vi "Emballage_NumSerie.vi"(8 "Error in":errorcluster caption="Error in (no error)", 11 "Tableau n° valves":string[](array[string])) -> (0 "Error out":errorcluster)   [LabVIEW 2020]
uses:
  Modules/FS/60_FS_Controles/60_FS_SetGet.ctl
panel:
  # "Veuillez patienter\npendant la création des fichiers \"Numéros de Série\"\nMERCI"
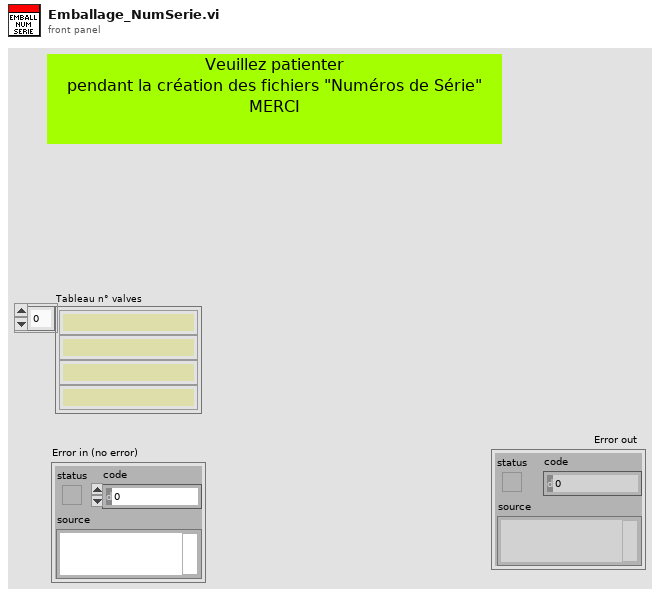
[diagram p1: front panel]
types:
  T1 = typedef "60_FS_SetGet.ctl" = enum16{"set", "get"}
  T2 = typedef "Emballage_BDD_param_Produit.ctl" = cluster{"No_Valve_FAS":string, "suffixe":string, "designation":string, "indice_produit":string, "code_barre_fixe":string, "affiche_code_barre_client":string, "affiche_no_client":string, "Nb_vlve_par_carton":u16, "melange_des_lots_possible":string, "id_article":string, "Indice_Rev":string, "Famille":string, "date":string, "code_barre_fixe_Fin":string, "Longeur_No_Serie":string}
  T3 = typedef "DATA commande.ctl" = cluster{"n°article FAS":string, "n° cmde FAS":string, "quantité cmde":string, "ID LIG cmde":string, "n° cmde client":string, "nom client":string, "n° article client":string, "indice revision client":string, "société de facturation":string, "langue a utiliser":string}
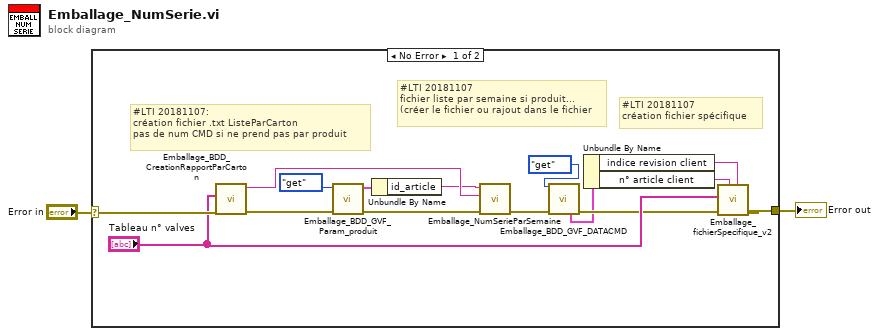
[diagram p0: block diagram]
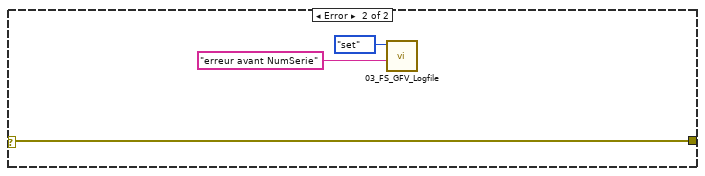
[diagram p2: hidden frame]
diagram:
  n1 = case shown="No Error" "Error in" {
    selector: "Error in" -> [w10 w18]
    tunnel: [w9 w18] -> w1
    frame No Error {
      # "#LTI 20181107\ncréation fichier spécifique"
      # "#LTI 20181107\nfichier liste par semaine si produit...\n(créer le fichier ou rajout dans le fichier"
      # "#LTI 20181107:\ncréation fichier .txt ListeParCarton\npas de num CMD si ne prend pas par produit"
      n2 = call "Emballage_BDD_CreationRapportParCarton.vi"("error in (no error)"=w10, "Tableau n° valves"="Tableau n° valves") -> ("error out"=w12:errorcluster, "chaîne concaténée"=w16:string)  [unwired: 6 in, 2 out]
      n3 = call "Emballage_BDD_GVF_Param_produit.vi"("Error in"=w12, "Énum"=enum16{"set", "get"}."get") -> ("Error out"=w11:errorcluster, "CLS_param_produit"=w14:T2)  [unwired: 6 in, 2 out]
      n4 = Unbundle By Name(w14) -> ("id_article"=w13:string)
      n5 = call "Emballage_NumSerieParSemaine.vi"("Error in"=w11, "texte"=w16, "ID_ARTICLE"=w13) -> ("Error out"=w17:errorcluster)  [unwired: 8 in]
      n6 = call "Emballage_BDD_GVF_DATACMD.vi"("SetGet"=60_FS_SetGet."get", "Error in"=w17) -> ("DATA cmde OUT"=w5:T3, "Error out"=w7:errorcluster)  [unwired: 6 in, 6 out]
      n7 = Unbundle By Name(w5) -> ("indice revision client"=w3:string, "n° article client"=w4:string)
      n8 = call "Emballage_fichierSpecifique_v2.vi"("Indice Rev. Client"=w3, "N° article client"=w4, "error in (no error)"=w7, "Tableau n° valves"="Tableau n° valves") -> ("error out"=w9:errorcluster)  [unwired: 7 in]
    }
    frame Error {
      n9 = call "03_FS_GFV_Logfile.vi"("Chaîne"="erreur avant NumSerie", "States"=60_FS_SetGet."set") -> ()  [unwired: 8 in, 2 out]
    }
  }
  "Error out" <- w1
